vi "PhotonPipelineResult_New.vi"(8 "PhotonMultiTargetPNPResult":T2={"PhotonPNPResult"={"IsPresent"=FALSE, "bestReprojErr"=0.0, "altReprojErr"=0.0, "ambiguity"=0.0, "Best"={"TRANSLATION3D"={"X"=0.0, "Y"=0.0, "Z"=0.0}, "ROTATION3D"={"Q_quaternion"={"R"=1.0, "V"=[0.0, 0.0, 0.0]}}, "XF"=FALSE}, "Alt"={"TRANSLATION3D"={"X"=0.0, "Y"=0.0, "Z"=0.0}, "ROTATION3D"={"Q_quaternion"={"R"=1.0, "V"=[0.0, 0.0, 0.0]}}, "XF"=FALSE}}, "FiducialIDsUsed"=[]} {"PhotonPNPResult"."Alt"."TRANSLATION3D"."Z" format="%14.3f"; "PhotonPNPResult"."Alt"."TRANSLATION3D"."Y" format="%14.3f"; "PhotonPNPResult"."Alt"."TRANSLATION3D"."X" format="%14.3f"; "PhotonPNPResult"."Best"."TRANSLATION3D"."Z" format="%14.3f"; "PhotonPNPResult"."Best"."TRANSLATION3D"."Y" format="%14.3f"; "PhotonPNPResult"."Best"."TRANSLATION3D"."X" format="%14.3f"}, 9 "TrackedTargets":T8[](array[typedef]) {"AltCameraToTarget"."TRANSLATION3D"."Z" format="%14.3f"; "AltCameraToTarget"."TRANSLATION3D"."Y" format="%14.3f"; "AltCameraToTarget"."TRANSLATION3D"."X" format="%14.3f"; "BestCameraToTarget"."TRANSLATION3D"."Z" format="%14.3f"; "BestCameraToTarget"."TRANSLATION3D"."Y" format="%14.3f"; "BestCameraToTarget"."TRANSLATION3D"."X" format="%14.3f"}, 11 "Latency_Millis":dbl) -> (3 "PhotonPipelineResult_REF":T1)   [LabVIEW 2019, in "PhotonVisionLib.lvlib"]
doc: "Create a new PhotonPipelineResult cluster.\n\nInputs:\n - Latency_Millis -- Latency, milliseconds\n - TrackedTargets -- Array of TracedTarget clusters\n - PhotonMultiTargetPNPResult - Multi Target Result.\n\nOutputs:\n - PipelineResult -- Parsed PipelineResult cluster."
uses:
  PhotonVisionLib.lvlib
  TypeDef/PhotonPipelineResultType.ctl
  TypeDef/PhotonTrackedTargetType.ctl
  TypeDef/TargetCornerType.ctl
  <vilib>/Rock Robotics/WPI/ThirdParty/JAS_Junk/TrajLib/TypeDef/QUATERNION.ctl
  <vilib>/Rock Robotics/WPI/ThirdParty/JAS_Junk/TrajLib/Trajectory_Library.lvlib
  <vilib>/Rock Robotics/WPI/ThirdParty/JAS_Junk/TrajLib/TypeDef/ROTATION3D.ctl
  <vilib>/Rock Robotics/WPI/ThirdParty/JAS_Junk/TrajLib/TypeDef/TRANSLATION3D.ctl
  <vilib>/Rock Robotics/WPI/ThirdParty/JAS_Junk/TrajLib/TypeDef/TRANSFORM3D.ctl
  TypeDef/PhotonPNPResultType.ctl
  TypeDef/PhotonMultiTargetPNPResultType.ctl
  Ref/PhotonPipelineResult_REF.ctl
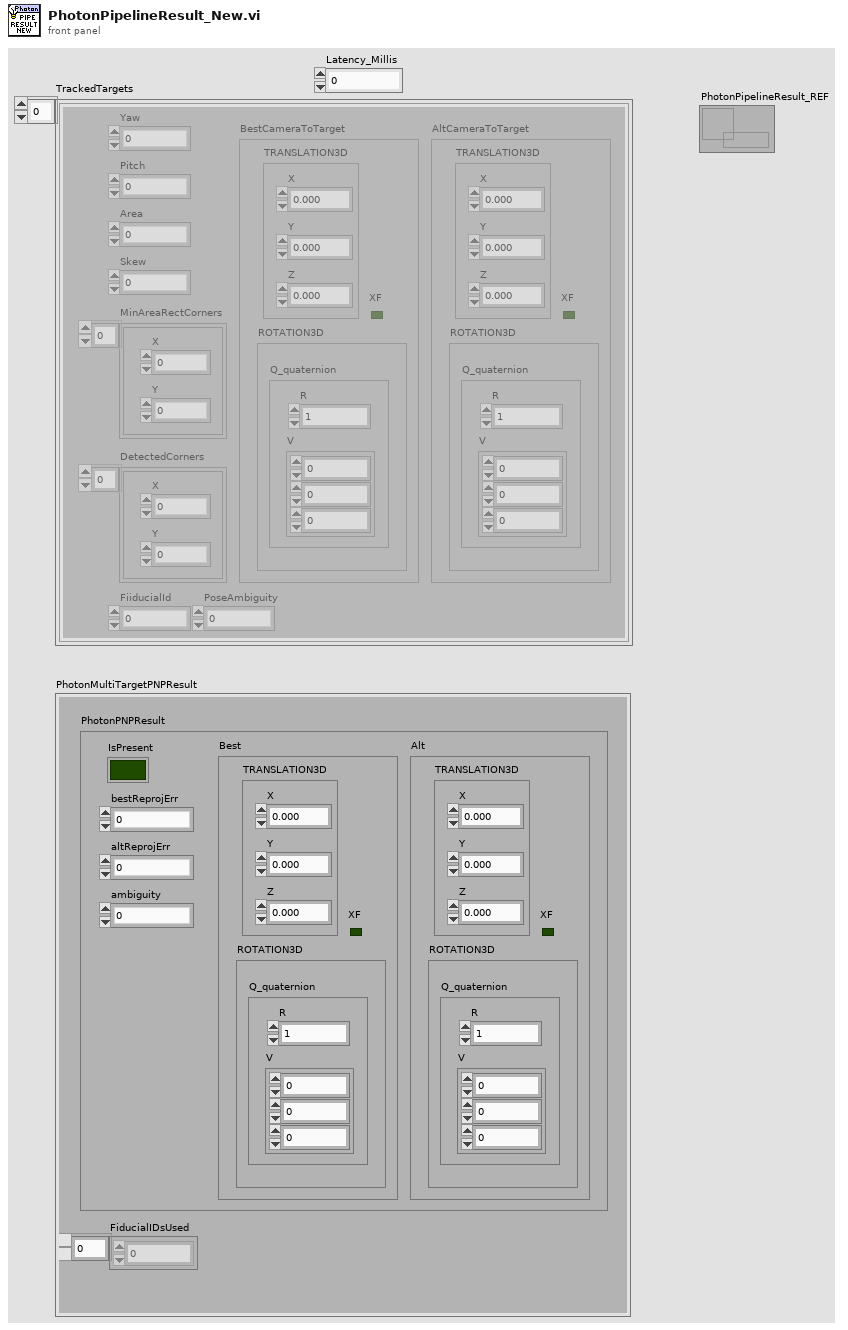
[diagram p1: front panel]
types:
  T1 = typedef "PhotonVisionLib.lvlib/PhotonPipelineResult_REF.ctl" = refnum<data-value>
  T2 = typedef "PhotonVisionLib.lvlib/PhotonMultiTargetPNPResultType.ctl" = cluster{"PhotonPNPResult":T3, "FiducialIDsUsed":i16[]}
  T3 = typedef "PhotonVisionLib.lvlib/PhotonPNPResultType.ctl" = cluster{"IsPresent":bool, "bestReprojErr":dbl, "altReprojErr":dbl, "ambiguity":dbl, "Best":T4, "Alt":T4}
  T4 = typedef "Trajectory_Library.lvlib/TRANSFORM3D.ctl" = cluster{"TRANSLATION3D":T5, "ROTATION3D":T6, "XF":bool}
  T5 = typedef "Trajectory_Library.lvlib/TRANSLATION3D.ctl" = cluster{"X":dbl, "Y":dbl, "Z":dbl}
  T6 = typedef "Trajectory_Library.lvlib/ROTATION3D.ctl" = cluster{"Q_quaternion":T7}
  T7 = typedef "Trajectory_Library.lvlib/QUATERNION.ctl" = cluster{"R":dbl, "V":dbl[]}
  T8 = typedef "PhotonVisionLib.lvlib/PhotonTrackedTargetType.ctl" = cluster{"Yaw":dbl, "Pitch":dbl, "Area":dbl, "Skew":dbl, "MinAreaRectCorners":T9[], "BestCameraToTarget":T4, "FiiducialId":i32, "AltCameraToTarget":T4, "PoseAmbiguity":dbl, "DetectedCorners":T9[]}
  T9 = typedef "PhotonVisionLib.lvlib/TargetCornerType.ctl" = cluster{"X":dbl, "Y":dbl}
  T10 = typedef "PhotonVisionLib.lvlib/PhotonPipelineResultType.ctl" = cluster{"TargetCount":i32, "Latency_MilliSec":dbl, "Targets":T8[], "TimeStampSec":dbl, "PhotonMultiTargetPNPResult":T2}
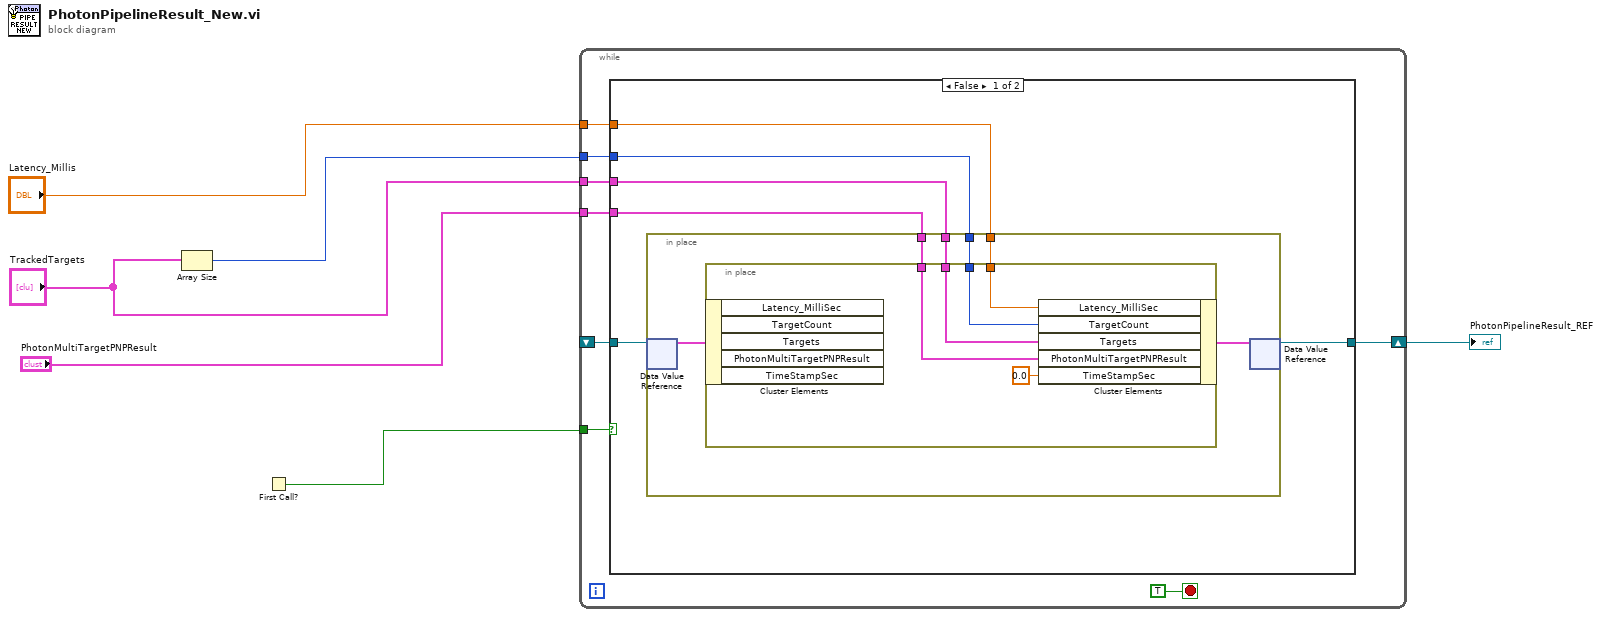
[diagram p0: block diagram]
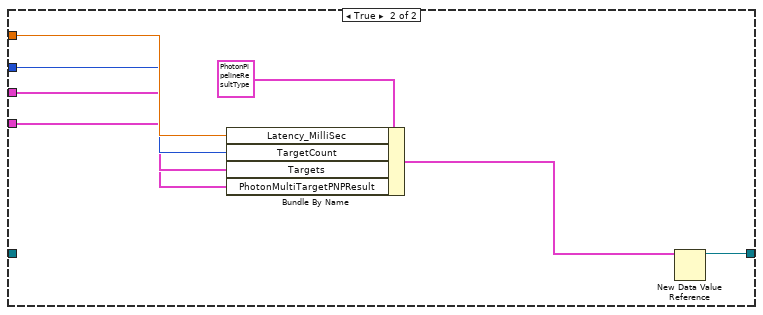
[diagram p2: hidden frame]
diagram:
  n1 = Array Size(array="TrackedTargets") -> (size(s)=w4:i32)
  n2 = First Call?() -> (First Call?: T/F=w6:bool)
  n3 = while {
    tunnel: w6 -> [w13]
    shift-right: [w14] -> w1
    shift-left: _ -> [w11]
    tunnel: "Latency_Millis" -> [w10]
    tunnel: w4 -> [w9]
    tunnel: "TrackedTargets" -> [w8]
    tunnel: "PhotonMultiTargetPNPResult" -> [w7]
    stop <- TRUE stop-if-true
    n4 = case shown="False" w13 {
      tunnel: [w19 w38] -> w14
      tunnel: w11 -> [w20 _]
      tunnel: w10 -> [w18 w36]
      tunnel: w9 -> [w17 w35]
      tunnel: w8 -> [w16 w34]
      tunnel: w7 -> [w15 w33]
      frame False {
        n5 = in-place {
          in-place-border: w18 -> [w26]
          in-place-border: w17 -> [w25]
          in-place-border: w16 -> [w24]
          in-place-border: w15 -> [w23]
          n6 = in-place-dvr #1(w20) -> (w21:T10)  [unwired: 1 out]
          n7 = in-place {
            in-place-border: w26 -> [w31]
            in-place-border: w25 -> [w30]
            in-place-border: w24 -> [w29]
            in-place-border: w23 -> [w28]
            n8 = in-place-cluster #2(w21) -> ()  [unwired: 5 out]
            n9 = in-place-cluster #2("Latency_MilliSec"=w31, "TargetCount"=w30, "Targets"=w29, "PhotonMultiTargetPNPResult"=w28, "TimeStampSec"=0.0) -> (w22:T10)
          }
          n10 = in-place-dvr #1(w22) -> (w19:refnum<data-value>)  [unwired: 1 out]
        }
      }
      frame True {
        n11 = Bundle By Name(cluster=T10 {"TargetCount"=0, "Latency_MilliSec"=0.0, "Targets"=[], "TimeStampSec"=0.0, "PhotonMultiTargetPNPResult"={"PhotonPNPResult"={"IsPresent"=FALSE, "bestReprojErr"=0.0, "altReprojErr"=0.0, "ambiguity"=0.0, "Best"={"TRANSLATION3D"={"X"=0.0, "Y"=0.0, "Z"=0.0}, "ROTATION3D"={"Q_quaternion"={"R"=1.0, "V"=[0.0, 0.0, 0.0]}}, "XF"=FALSE}, "Alt"={"TRANSLATION3D"={"X"=0.0, "Y"=0.0, "Z"=0.0}, "ROTATION3D"={"Q_quaternion"={"R"=1.0, "V"=[0.0, 0.0, 0.0]}}, "XF"=FALSE}}, "FiducialIDsUsed"=[]}} ("PhotonPipelineResult"), "Latency_MilliSec"=w36, "TargetCount"=w35, "Targets"=w34, "PhotonMultiTargetPNPResult"=w33) -> (w32:T10)
        n12 = New Data Value Reference(data value=w32) -> (data value reference=w38:refnum<data-value>)  [unwired: 1 in, 1 out]
      }
    }
  }
  "PhotonPipelineResult_REF" <- w1
